vi "demo.vi"() -> ()   [LabVIEW 2019]
uses:
  C:/Users/huang/Desktop/MIL LITE 10/64/Matrox Imaging/MIL/MIL.NET/Matrox.MatroxImagingLibrary.v3.5.dll
  64/Matrox Imaging/MIL/MIL.NET/Matrox.MatroxImagingLibrary.v3.5.dll
panel:
  out "number 2":i32
  out "number":i32
  out "UserArrayPtr":u16[](array[numeric])
  in  "停止":bool
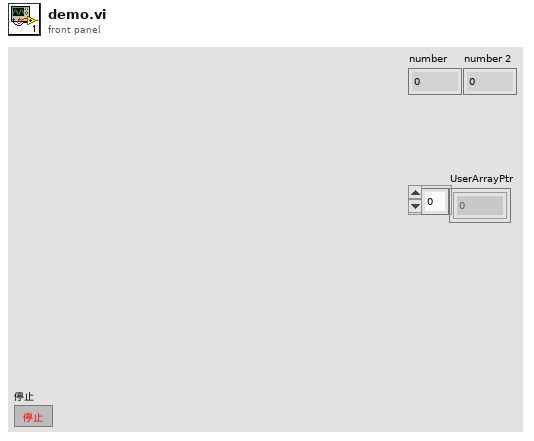
[diagram p1: front panel]
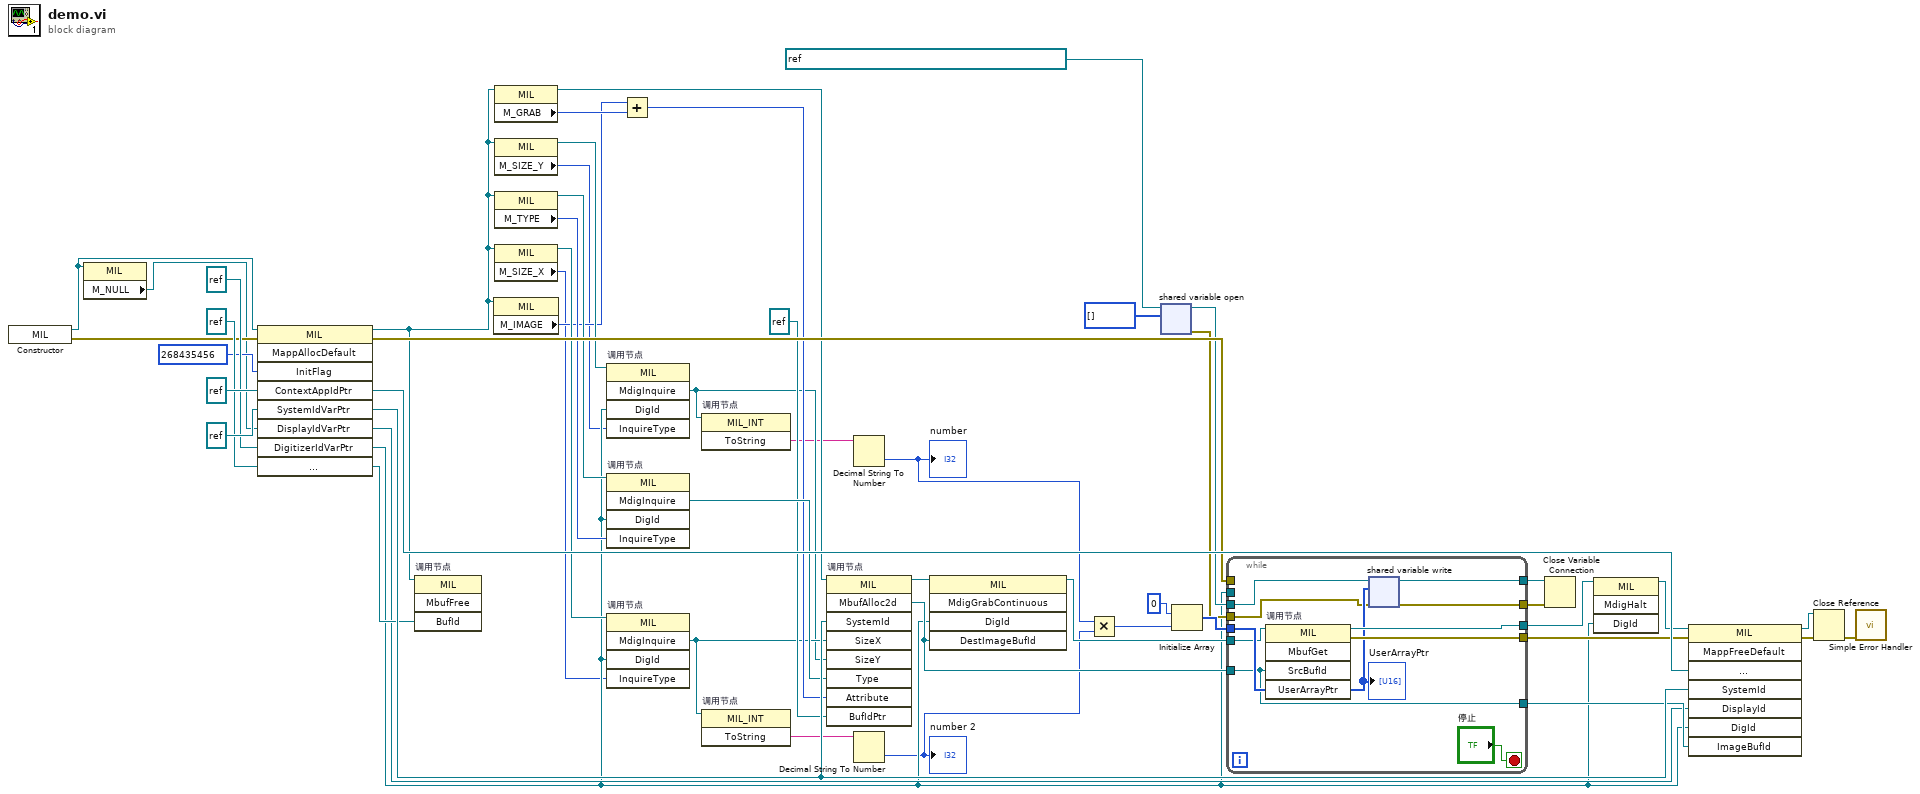
[diagram p0: block diagram]
diagram:
  n1 = constructor class="MIL"() -> (reference out=w21:refnum<k24>, error out=w41:errorcluster)  [unwired: 3 in, 1 out]
  n2 = property class="MIL"(reference=w21) -> ("M_NULL"=w20:refnum<k24>)  [unwired: 1 in, 2 out]
  n3 = invoke on="调用节点" class="MIL" method="MappAllocDefault"(reference=w21, error in=w41, "InitFlag"=i64 268435456, "ContextAppIdPtr"=refnum<k24> refnum, "SystemIdVarPtr"=refnum<k24> refnum, "DisplayIdVarPtr"=w20, "DigitizerIdVarPtr"=refnum<k24> refnum, "ImageIdVarPtr"=refnum<k24> refnum) -> (reference out=w1:refnum<k24>, error out=w45:errorcluster, "ContextAppIdPtr"=w48:refnum<k24>, "SystemIdVarPtr"=w38:refnum<k24>, "DisplayIdVarPtr"=w12:refnum<k24>, "DigitizerIdVarPtr"=w11:refnum<k24>, "ImageIdVarPtr"=w18:refnum<k24>)  [unwired: 1 in, 2 out]
  n4 = invoke on="调用节点" class="MIL" method="MbufFree"(reference=w1, "BufId"=w18) -> ()  [unwired: 2 in, 4 out]
  n5 = property class="MIL"(reference=w1) -> ("M_IMAGE"=w30:i32)  [unwired: 1 in, 2 out]
  n6 = property class="MIL"(reference=w1) -> (reference out=w28:refnum<k24>, "M_GRAB"=w31:i32)  [unwired: 1 in, 1 out]
  n7 = property class="MIL"(reference=w1) -> (reference out=w37:refnum<k24>, "M_SIZE_Y"=w9:i32)  [unwired: 1 in, 1 out]
  n8 = property class="MIL"(reference=w1) -> (reference out=w35:refnum<k24>, "M_TYPE"=w34:i32)  [unwired: 1 in, 1 out]
  n9 = property class="MIL"(reference=w1) -> (reference out=w36:refnum<k24>, "M_SIZE_X"=w10:i32)  [unwired: 1 in, 1 out]
  n10 = invoke on="调用节点" class="MIL" method="MdigInquire"(reference=w37, "DigId"=w11, "InquireType"=w9) -> ("MdigInquire"=w4:refnum<k24>)  [unwired: 2 in, 4 out]
  n11 = invoke on="调用节点" class="MIL" method="MdigInquire"(reference=w35, "DigId"=w11, "InquireType"=w34) -> ("MdigInquire"=w33:refnum<k24>)  [unwired: 2 in, 4 out]
  n12 = invoke on="调用节点" class="MIL" method="MdigInquire"(reference=w36, "DigId"=w11, "InquireType"=w10) -> ("MdigInquire"=w7:refnum<k24>)  [unwired: 2 in, 4 out]
  n13 = Add(x=w30, y=w31) -> (x+y=w29:i32)
  n14 = invoke on="调用节点" class="MIL_INT" method="ToString"(reference=w4) -> ("ToString"=w3:string)  [unwired: 2 in, 2 out]
  n15 = invoke on="调用节点" class="MIL_INT" method="ToString"(reference=w7) -> ("ToString"=w6:string)  [unwired: 2 in, 2 out]
  n16 = invoke on="调用节点" class="MIL" method="MbufAlloc2d"(reference=w28, "SystemId"=w38, "SizeX"=w7, "SizeY"=w4, "Type"=w33, "Attribute"=w29, "BufIdPtr"=refnum<k24> refnum) -> (reference out=w17:refnum<k24>, "MbufAlloc2d"=w15:refnum<k24>)  [unwired: 2 in, 7 out]
  n17 = Decimal String To Number(string=w3) -> (number=w2:i32)  [unwired: 2 in, 1 out]
  "number" <- w2
  n18 = Decimal String To Number(string=w6) -> (number=w5:i32)  [unwired: 2 in, 1 out]
  "number 2" <- w5
  n19 = invoke on="调用节点" class="MIL" method="MdigGrabContinuous"(reference=w17, "DigId"=w11, "DestImageBufId"=w15) -> (reference out=w16:refnum<k24>)  [unwired: 2 in, 4 out]
  n20 = Multiply(x=w2, y=w5) -> (x*y=w8:i32)
  n21 = shared-variable-open(refnum<k21> "ni.var.psp://my computer/sharevariable/buf" ("shared variable refnum in"), u16[] []) -> (w26:refnum<k21>, w23:errorcluster)  [unwired: 2 in]
  n22 = Initialize Array(u16 0 ("element"), w8) -> (w39:u16[])
  n23 = while {
    tunnel: w11 -> [_]
    tunnel: [w62] -> w14
    tunnel: w45 -> [_]
    tunnel: [w61] -> w44
    tunnel: w39 -> [w60]
    tunnel: w15 -> [w54]
    tunnel: w26 -> [w59]
    tunnel: [w57] -> w25
    tunnel: [w56] -> w24
    tunnel: w23 -> [w55]
    tunnel: [w54] -> w19
    tunnel: w16 -> [w53]
    stop <- "停止" stop-if-true
    n24 = invoke on="调用节点" class="MIL" method="MbufGet"(reference=w53, "SrcBufId"=w54, "UserArrayPtr"=w60) -> (reference out=w62:refnum<k24>, error out=w61:errorcluster, "UserArrayPtr"=w58:u16[])  [unwired: 2 in, 2 out]
    "UserArrayPtr" <- w58
    n25 = shared-variable-write(w59, w55, w58) -> (w57:refnum<k21>, w56:errorcluster)
  }
  n26 = Close Variable Connection(8:w24, 11:w25) -> ()  [unwired: 1 out]
  n27 = invoke on="调用节点" class="MIL" method="MdigHalt"(reference=w14, "DigId"=w11) -> (reference out=w13:refnum<k24>)  [unwired: 2 in, 3 out]
  n28 = invoke on="调用节点" class="MIL" method="MappFreeDefault"(reference=w13, error in=w44, "ApplicationId"=w48, "SystemId"=w38, "DisplayId"=w12, "DigId"=w11, "ImageBufId"=w19) -> (reference out=w46:refnum<k24>, error out=w43:errorcluster)  [unwired: 1 in, 6 out]
  n29 = Close Reference(reference=w46, error in (no error)=w43) -> (error out=w42:errorcluster)
  n30 = call <vilib>:"Simple Error Handler.vi"("error in (no error)"=w42) -> ()  [unwired: 4 in, 5 out]
